vi "interop.vi"() -> ()   [LabVIEW 2022 SP3]
uses:
  return value.ctl
  <vilib>/Utility/error.llb/DialogType.ctl
  cluster.ctl
  cluster 2.ctl
panel:
  out "Array":dbl[][](array[numeric])
  out "return array":T1[](array[typedef])
  out "return value":T1
  in  "Python version":string="3.9"
  out "String":string
  in  "module path":path=path "R:/work/FS-call-a-python-function-from-LabVIEW/interop/interop.py"
  in  "error in":errorcluster
  out "error out":errorcluster
  in  "Python path":path=path "C:/Users/Mikio Fukushima/AppData/Local/Programs/Python/Python39/python.exe"
  # "pythonスクリプトのパスに2バイトコードを含めるとエラーになるので注意。"
  # "LabVIEW.iniに\nShowConsoleForPythonNode=TRUE\nを追加すると、Pythonノード実行時にコンソールが開いて標準出力を見る事が出来る。"
  # "Pythonノードを使用したLabVIEWへの/LabVIEWからのPythonデータ構造の受け渡し\nhttps://knowledge.ni.com/KnowledgeArticleDetails?id=kA03q000000oyaHCAQ&l=ja-JP"
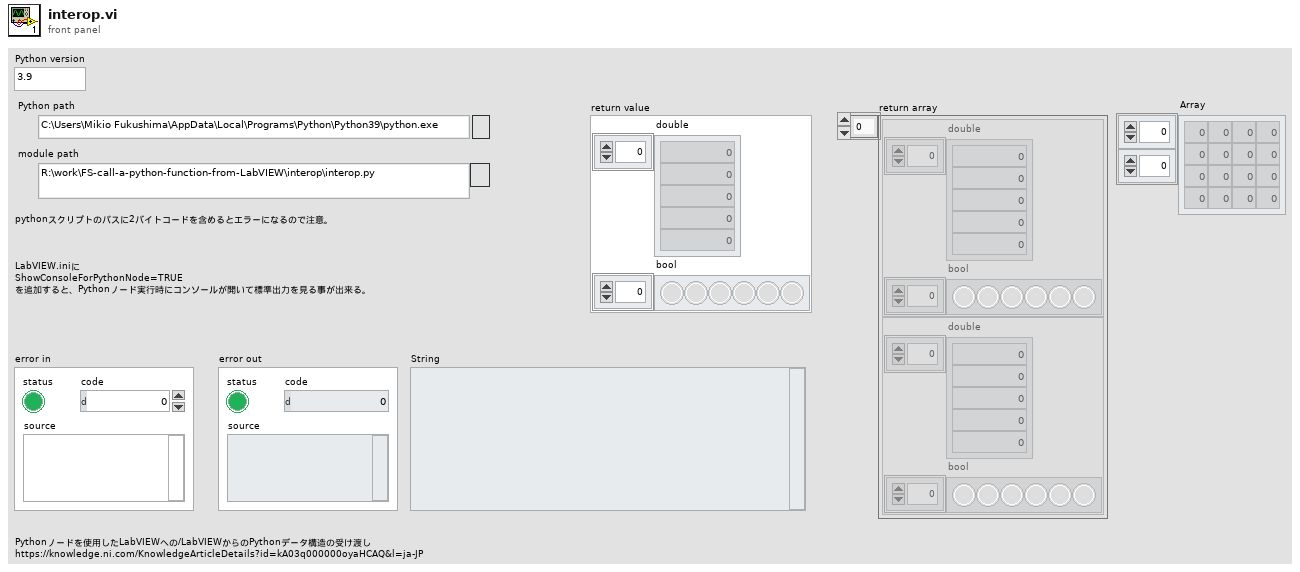
[diagram p1: front panel]
types:
  T1 = typedef "return value.ctl" = cluster{"double":dbl[], "bool":bool[]}
  T2 = typedef "cluster 2.ctl" = cluster{"Enum":enum16{"Item1", "Item2"}}
  T3 = typedef "cluster.ctl" = cluster{"double":dbl, "i32 array":i32[], "String":string, "Cluster 2":T2}
  T4 = typedef "DialogType.ctl" = u16
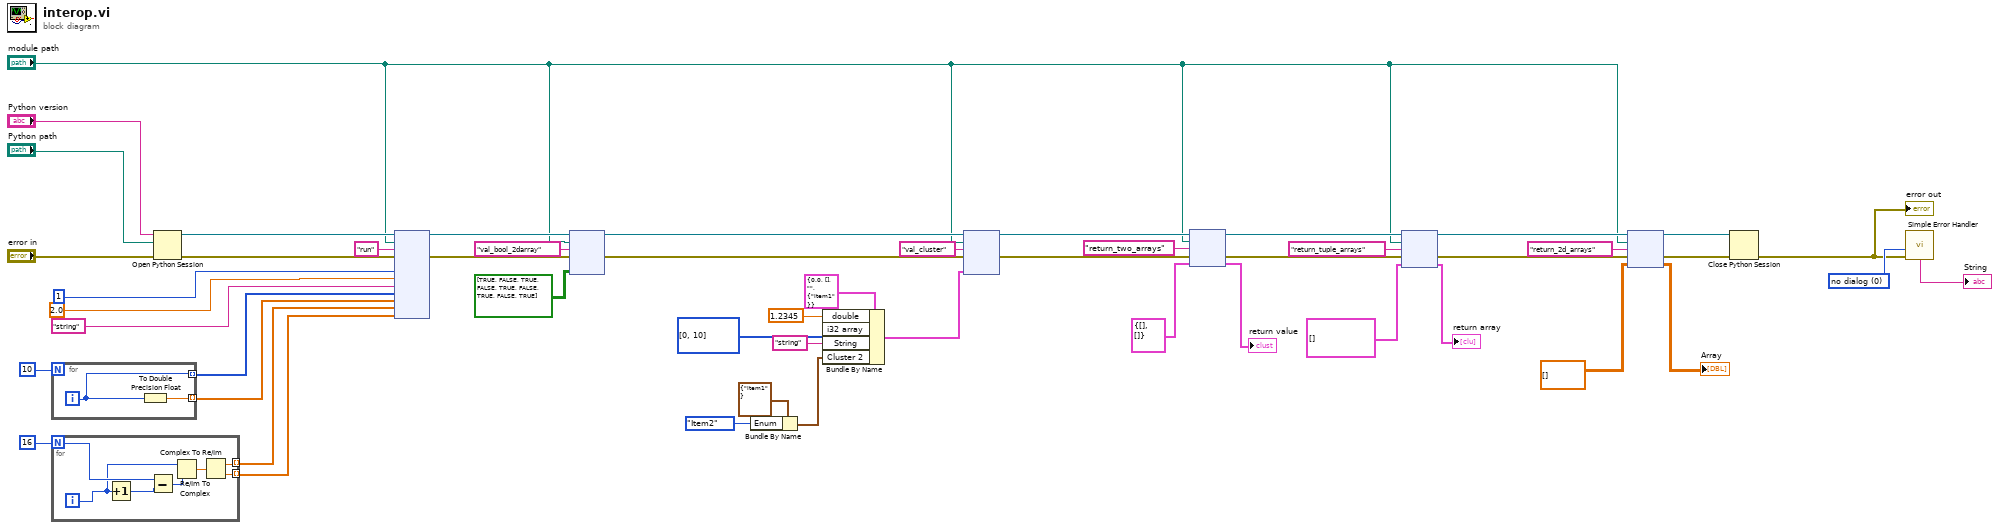
[diagram p0: block diagram]
diagram:
  w47 = T4 0 items=["no dialog", "OK message", "continue or stop message", "OK message + warnings", "continue/stop + warnings"] ("type of dialog (OK msg:1)")
  n1 = for {
    N: 10 -> [_]
    tunnel: [w53] -> w40 mode=indexing
    tunnel: [w52] -> w41 mode=indexing
    i -> [w53]
    n2 = To Double Precision Float(number=w53) -> (double precision float=w52:dbl)
  }
  n3 = for {
    N: 16 -> [w57]
    tunnel: [w60] -> w38 mode=indexing
    tunnel: [w59] -> w39 mode=indexing
    i -> [w56]
    n4 = Increment(x=w56) -> (x+1=w54:i32)
    n5 = Subtract(x=w57, y=w54) -> (x-y=w55:i32)
    n6 = Re/Im To Complex(1:w55, 2:w56) -> (0:w58:cdb)
    n7 = Complex To Re/Im(x + iy=w58) -> (x=w60:dbl, y=w59:dbl)
  }
  n8 = Open Python Session(python version="Python version", python path="Python path", 3:"error in") -> (session out=w50:refnum<k35>, error out=w49:errorcluster)
  n9 = node(w50, "module path", "run" ("function name"), w49, 1, 2.0, "string", w40, w41, w38, w39) -> (w11:refnum<k35>, w8:errorcluster)  [unwired: 9 in, 2 out]
  n10 = node(w11, "module path", "val_bool_2darray" ("function name"), w8, bool[][] [[TRUE, FALSE, TRUE], [FALSE, TRUE, FALSE], [TRUE, FALSE, TRUE]]) -> (w7:refnum<k35>, w6:errorcluster)  [unwired: 3 in, 2 out]
  n11 = Bundle By Name(cluster=T2 {"Enum"=enum."Item1"} ("Cluster 2"), "Enum"=enum16{"Item1", "Item2"}."Item2") -> (w31:T2)
  n12 = Bundle By Name(cluster=T3 {"double"=0.0, "i32 array"=[], "String"="", "Cluster 2"={"Enum"=enum."Item1"}} ("Cluster"), "double"=1.2345, "i32 array"=i32[] [0, 10], "String"="string", "Cluster 2"=w31) -> (w1:T3)
  n13 = node(w7, "module path", "val_cluster" ("function name"), w6, w1) -> (w4:refnum<k35>, w5:errorcluster)  [unwired: 3 in, 2 out]
  n14 = node(w4, "module path", "return_two_arrays" ("function name"), w5, T1 {"double"=[], "bool"=[]} ("return value")) -> (w23:refnum<k35>, w22:errorcluster, →"return value":T1)  [unwired: 2 out]
  n15 = node(w23, "module path", "return_tuple_arrays" ("function name"), w22, T1[] []) -> (w17:refnum<k35>, w15:errorcluster, →"return array":T1[])  [unwired: 2 out]
  n16 = node(w17, "module path", "return_2d_arrays" ("function name"), w15, dbl[][] []) -> (w16:refnum<k35>, w14:errorcluster, →"Array":dbl[][])  [unwired: 2 out]
  n17 = Close Python Session(session in=w16, error in=w14) -> (11:w24:errorcluster)
  "error out" <- w24
  n18 = call <vilib>:"Simple Error Handler.vi"("type of dialog (OK msg:1)"=w47, "error in (no error)"=w24) -> ("message"=→"String":string)  [unwired: 3 in, 4 out]
